vi "EEI EXP Trial2.vi"(2 "Fahrenheit 2":dbl, 3 "Celcius 1":dbl) -> (0 "Celcuis 2":dbl, 1 "Fahrenheit 1":dbl)   [LabVIEW 2020]
panel:
  out "current time":timestamp
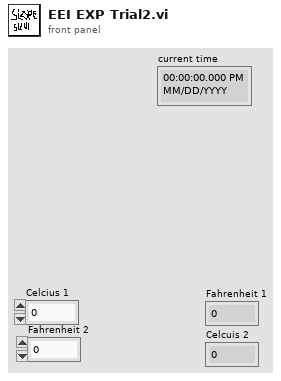
[diagram p1: front panel]
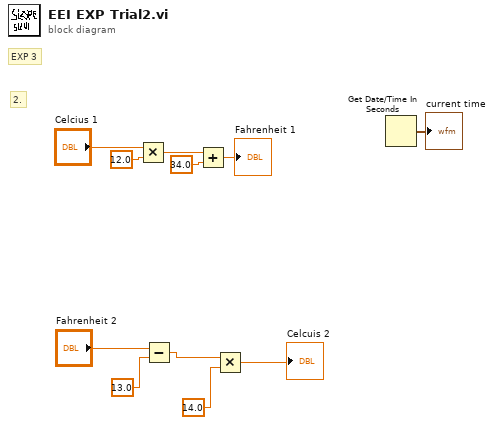
[diagram p0: block diagram]
diagram:
  # "2."
  # "EXP 3"
  n1 = Multiply(x="Celcius 1", y=12.0) -> (x*y=w9:dbl)
  n2 = Subtract(x="Fahrenheit 2", y=13.0) -> (x-y=w4:dbl)
  n3 = Add(x=w9, y=34.0) -> (x+y=→"Fahrenheit 1":dbl)
  n4 = Multiply(x=w4, y=14.0) -> (x*y=→"Celcuis 2":dbl)
  n5 = Get Date/Time In Seconds() -> (seconds since 1Jan1904=→"current time":timestamp)
